vi "Update Message Data.vi"(0 "Data In":string, 7 "Update Information":string, 11 "Error In":errorcluster) -> (4 "Data Out":string, 15 "Error Out":errorcluster)   [LabVIEW 2016, in "GEA2_Toolkit.lvlib"]
doc: "This VI can be used to modify the input data with the update information specified. The update information should contain all of the bits that you wish to be updated in the ERD. Just specify the bits you want to update (ex. 0=1) and put whether or not you want them to be True (1) or False (0). You can specify a range of bits by using the - command in between two numbers (ex. 0-7=1 would change bits 0, 1, 2, 3, 4, 5, 6, 7 to true). All spaces are removed from the update information at the beginning of this VI. The update information is converted to an array of strings by a comma delimiter. So, seperate your update information pieces by commas (Ex. if you wanted to make bits 0 and 10 false you could use the message: 0=0,10=0). Make sure you don't set the same bit twice or only the 2nd setting will ocurr (ex. 0=1,0=0 will only set bit 0 to false). If you were to write the following ERD data (00 01 02), byte 00 would be the byte 0 and contain bits 0-7, byte 01 would be byte 1 and contain bits 8-15, and byte 02 would be byte 2 and contain bits 16-23. For all bytes, the right-most bit is the first bit and the left-most bit is the last (Ex. For byte 00 being the hex value 0x01, bit 0 would be equal to 1 and would be the right-most bit (00000001)"
uses:
  library/GEA2_Toolkit.lvlib
  <vilib>/Utility/error.llb/whitespace.ctl
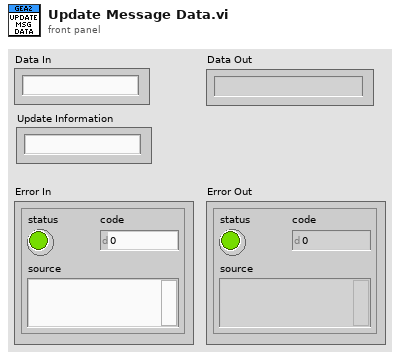
[diagram p1: front panel]
types:
  T1 = typedef "whitespace.ctl" = u16
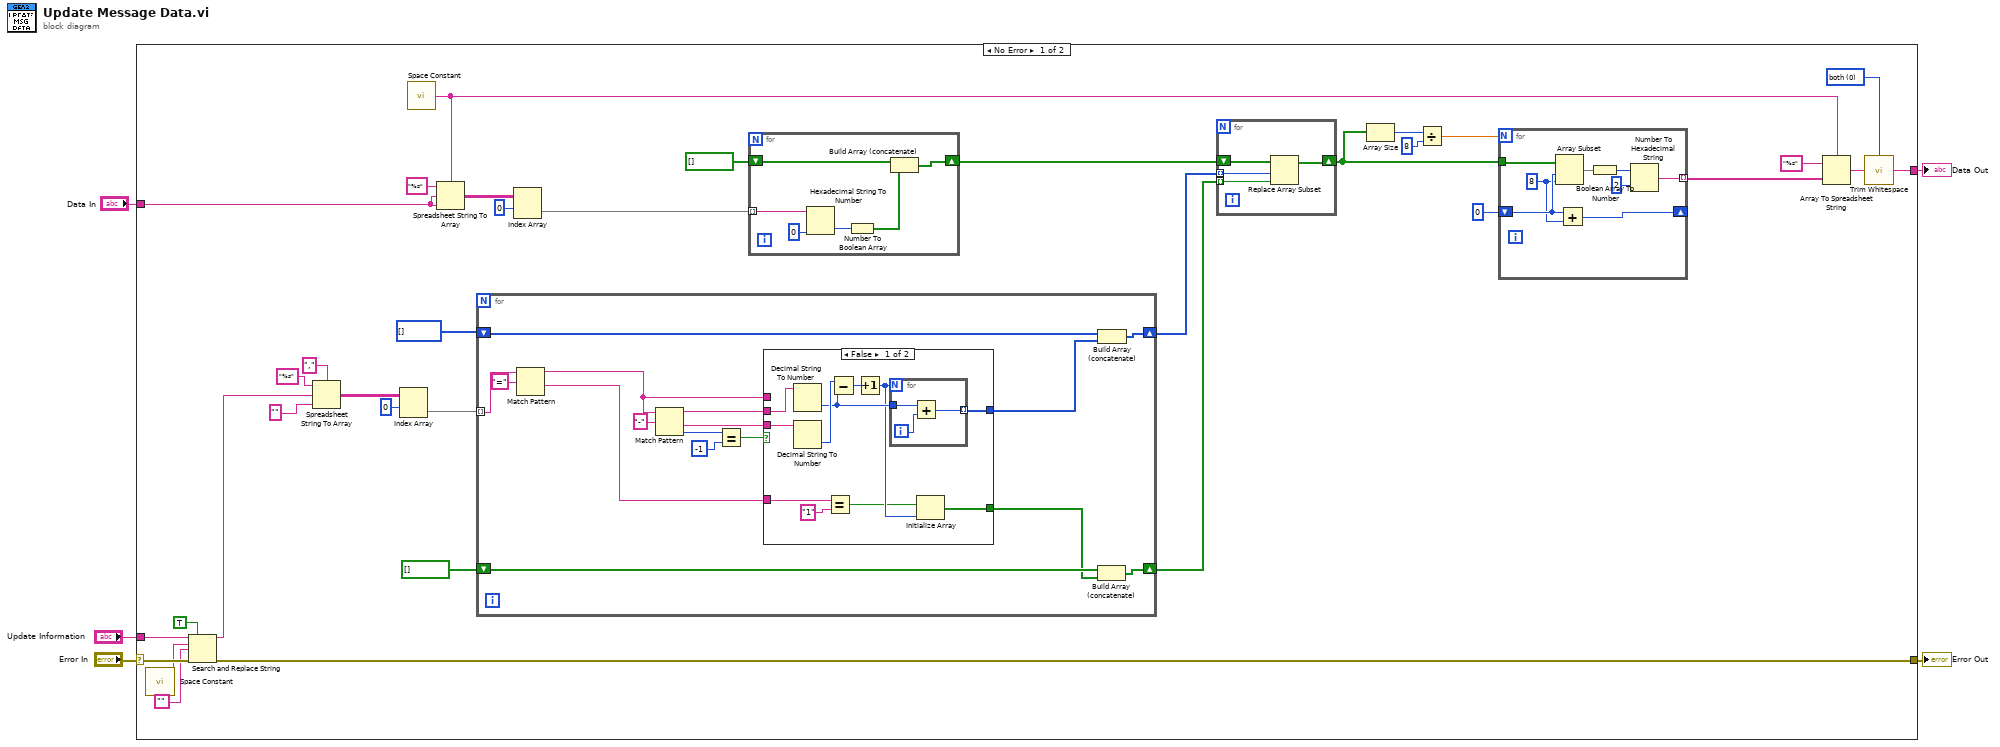
[diagram p0: block diagram]
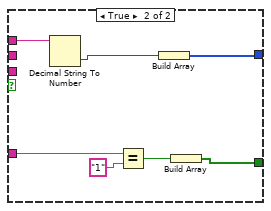
[diagram p2: hidden frame]
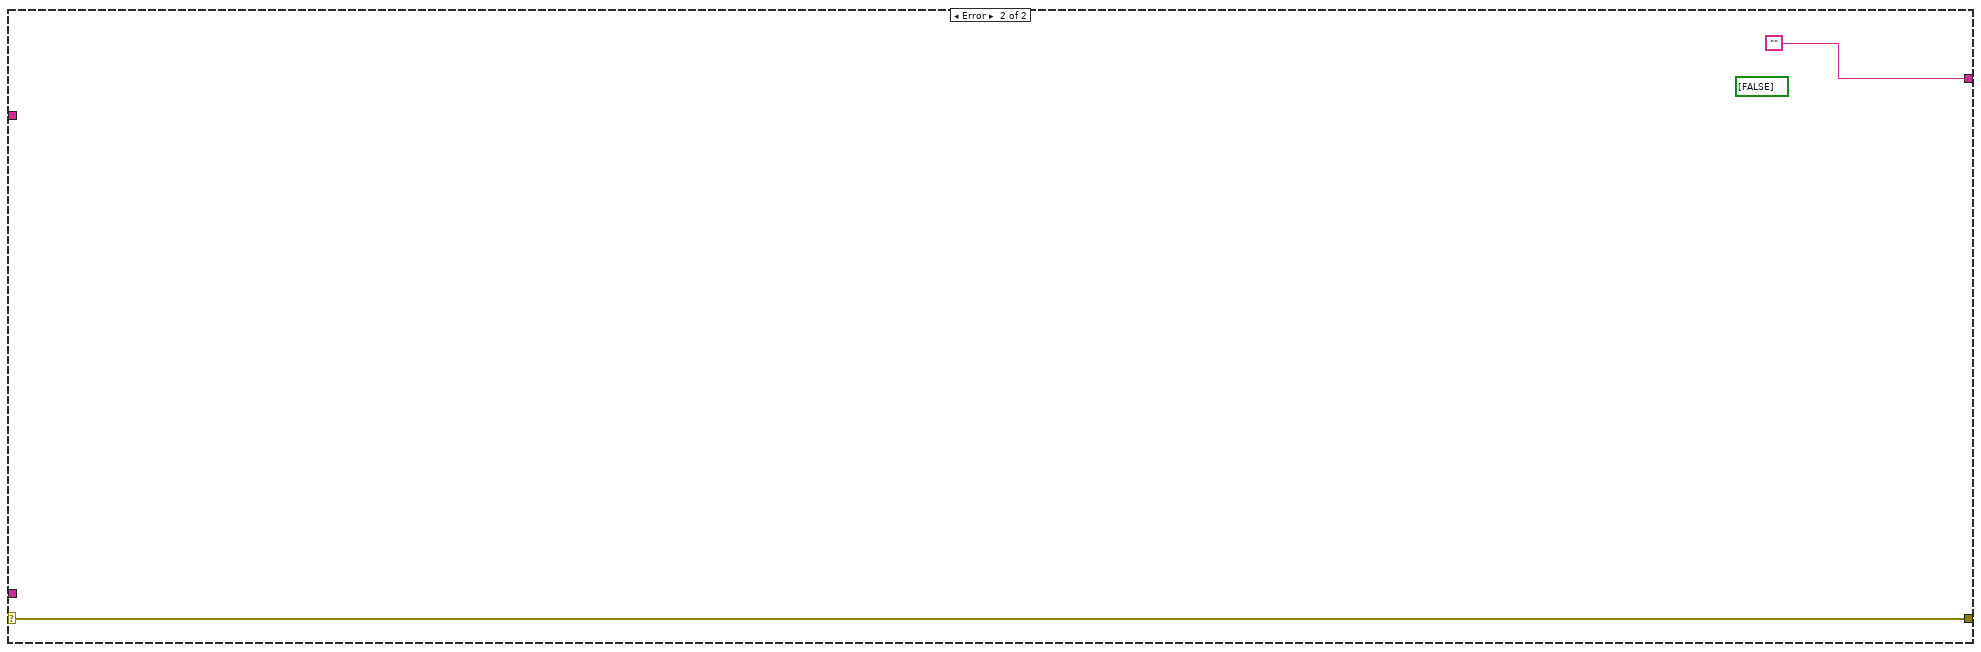
[diagram p3: hidden frame]
diagram:
  n1 = case shown="No Error" "Error In" {
    selector: "Error In" -> [w15 w97]
    tunnel: "Data In" -> [w37 _]
    tunnel: "Update Information" -> [w16 _]
    tunnel: [w14 w97] -> w2
    tunnel: [w8 ""] -> w1
    frame No Error {
      w6 = T1 0 items=["both", "start of string", "end of string"] ("location (both)")
      n2 = call <vilib>:"Space Constant.vi"() -> ("String"=w13:string)
      n3 = Search and Replace String(replace all?=TRUE ("replace all? (F)"), input string=w16, search string=w13, replace string="", error in=w15) -> (result string=w11:string, error out=w14:errorcluster)  [unwired: 3 in, 2 out]
      n4 = Spreadsheet String To Array(delimiter (Tab)=",", format string="%s", spreadsheet string=w11, array type (2D Dbl)="") -> (array=w32:string[][])
      n5 = Index Array(array=w32, index (row)=0) -> (element=w30:string[])  [unwired: 1 in]
      n6 = call <vilib>:"Space Constant.vi"() -> ("String"=w9:string)
      n7 = Spreadsheet String To Array(delimiter (Tab)=w9, format string="%s", spreadsheet string=w37, array type (2D Dbl)=w37) -> (array=w39:string[][])
      n8 = for {
        tunnel: w30 -> [w60] mode=indexing
        shift-right: [w62] -> w26
        shift-left: i32[] [] -> [w61]
        shift-right: [w53] -> w25
        shift-left: bool[] [] -> [w55]
        n9 = Match Pattern(string=w60, regular expression="=") -> (before substring=w58:string, after substring=w56:string)  [unwired: 1 in, 2 out]
        n10 = Match Pattern(string=w58, regular expression="-") -> (before substring=w64:string, after substring=w63:string, offset past match=w67:i32)  [unwired: 1 in, 1 out]
        n11 = Equal?(x=w67, y=-1) -> (x = y?=w65:bool)
        n12 = case shown="False" w65 {
          tunnel: w64 -> [w79 _]
          tunnel: w63 -> [w78 _]
          tunnel: w58 -> [_ w89]
          tunnel: [w75 w87] -> w57
          tunnel: w56 -> [w73 w85]
          tunnel: [w70 w83] -> w54
          frame False {
            n13 = Decimal String To Number(string=w79) -> (number=w76:i32)  [unwired: 2 in, 1 out]
            n14 = Decimal String To Number(string=w78) -> (number=w77:i32)  [unwired: 2 in, 1 out]
            n15 = Equal?(x=w73, y="1") -> (x = y?=w71:bool)
            n16 = Subtract(x=w77, y=w76) -> (x-y=w69:i32)
            n17 = Increment(x=w69) -> (x+1=w72:i32)
            n18 = for {
              N: w72 -> [_]
              tunnel: w76 -> [w82]
              tunnel: [w80] -> w75 mode=indexing
              i -> [w81]
              n19 = Add(x=w82, y=w81) -> (x+y=w80:i32)
            }
            n20 = Initialize Array(w71, w72) -> (w70:bool[])
          }
          frame True {
            n21 = Decimal String To Number(string=w89) -> (number=w88:i32)  [unwired: 2 in, 1 out]
            n22 = Equal?(x=w85, y="1") -> (x = y?=w84:bool)
            n23 = Build Array(w88) -> (w87:i32[])
            n24 = Build Array(w84) -> (w83:bool[])
          }
        }
        n25 = Build Array (concatenate)(w55, w54) -> (w53:bool[])
        n26 = Build Array (concatenate)(w61, w57) -> (w62:i32[])
      }
      n27 = Index Array(array=w39, index (row)=0) -> (element=w17:string[])  [unwired: 1 in]
      n28 = for {
        tunnel: w17 -> [w95] mode=indexing
        shift-right: [w93] -> w27
        shift-left: bool[] [] -> [w91]
        n29 = Hexadecimal String To Number(string=w95, default (0uL)=u8 0) -> (number=w94:u8)  [unwired: 1 in, 1 out]
        n30 = Number To Boolean Array(number=w94) -> (Boolean array=w90:bool[])
        n31 = Build Array (concatenate)(w91, w90) -> (w93:bool[])
      }
      n32 = for {
        tunnel: w26 -> [w52] mode=indexing
        tunnel: w25 -> [w50] mode=indexing
        shift-right: [w49] -> w21
        shift-left: w27 -> [w51]
        n33 = Replace Array Subset(array=w51, new element=w50, index=w52) -> (w49:bool[])
      }
      n34 = Array Size(array=w21) -> (size(s)=w24:i32)
      n35 = Divide(x=w24, y=8) -> (x/y=w22:dbl)
      n36 = for {
        N: w22 -> [_]
        tunnel: w21 -> [w48]
        shift-right: [w45] -> _
        shift-left: 0 ("length") -> [w47]
        tunnel: [w41] -> w18 mode=indexing
        w46 = 8 ("length")
        n37 = Array Subset(array=w48, index=w47, length=w46) -> (w44:bool[])
        n38 = Add(x=w47, y=w46) -> (x+y=w45:i32)
        n39 = Boolean Array To Number(Boolean array=w44) -> (number=w43:u32)
        n40 = Number To Hexadecimal String(1:i16 2 ("width (-)"), 2:w43) -> (0:w41:string)
      }
      n41 = Array To Spreadsheet String(delimiter (Tab)=w9, array=w18, 3:"%s" ("format string")) -> (spreadsheet string=w7:string)
      n42 = call <vilib>:"Trim Whitespace.vi"("string"=w7, "location (both)"=w6) -> ("trimmed string"=w8:string)
    }
    frame Error {
      (unwired) bool[] [FALSE]
    }
  }
  "Error Out" <- w2
  "Data Out" <- w1
